vi "未命名zzzz.vi"(11 "Slide引用句柄":refnum<vi>) -> (2 "颜色盒 2":u32(colorbox))   [LabVIEW 2015]
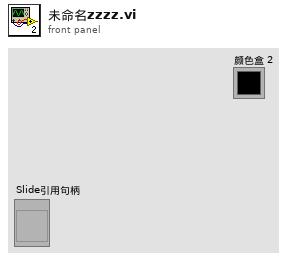
[diagram p1: front panel]
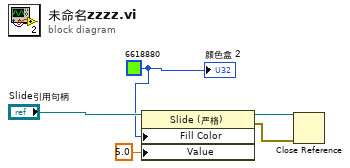
[diagram p0: block diagram]
diagram:
  w4 = u32 6618880 ("颜色盒")
  n1 = property class="Slide (严格)"(reference="Slide引用句柄", "Fill Color"=w4, "Value"=5.0 ("值")) -> (reference out=w2:refnum<vi>, error out=w1:errorcluster)  [unwired: 1 in]
  n2 = Close Reference(reference=w2, error in (no error)=w1) -> ()  [unwired: 1 out]
  "颜色盒 2" <- w4
